vi "Move Mirror.vi"(7 "Mono System # (0)":T1, 8 "error in (no error)":errorcluster, 9 "position (side/lateral)":enum16{"side (lateral)", "front (axial)"}(ring), 10 "mirror (exit)":enum16{"entrance", "exit"}(ring)=enum."exit", 11 "VISA resource name":refnum<visa-resource-name>) -> (0 "error out":errorcluster, 3 "VISA resource name out":refnum<visa-resource-name>)   [LabVIEW 2009, in "JY-SPEX-TRIAX.lvlib"]
doc: "Moves the entrance and exit mirrors to select either the front (axial) or side (lateral) positions, respectively."
uses:
  JY-SPEX-TRIAX.lvlib
  controls.llb/Monochromator System Number.ctl
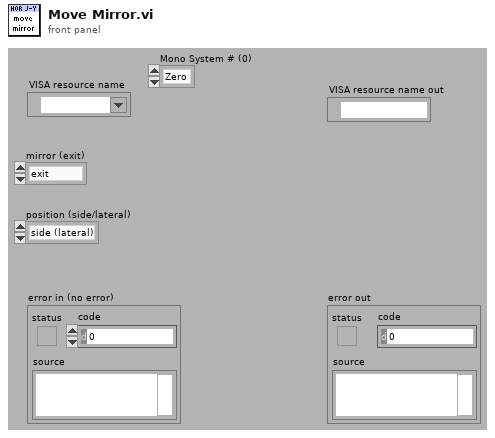
[diagram p1: front panel]
types:
  T1 = typedef "JY-SPEX-TRIAX.lvlib/Monochromator System Number.ctl" = enum16{"Zero", "One"}
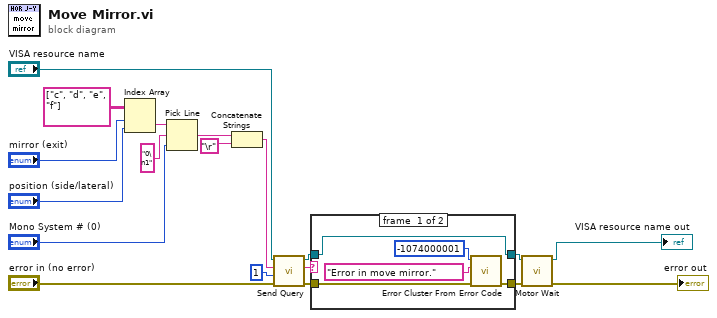
[diagram p0: block diagram]
diagram:
  n1 = Index Array(array=string[][] [["c", "d"], ["e", "f"]], index (row)="mirror (exit)", index (col)="position (side/lateral)") -> (element=w5:string)
  n2 = Pick Line(string ("")=w5, multi-line string="0\n1", line index="Mono System # (0)") -> (output string=w17:string)
  n3 = Concatenate Strings(w17, "\r") -> (w10:string)
  n4 = call "Send Query.vi"("error in (no error)"="error in (no error)", "byte count"=u32 1, "write buffer"=w10, "VISA resource name"="VISA resource name") -> ("error out"=w12:errorcluster, "read buffer"=w14:string, "VISA resource name out"=w13:refnum<visa-resource-name>)  [unwired: 5 out]
  n5 = case shown="Default" w14 {
    tunnel: w13 -> [w20 w26]
    tunnel: [w20 w26] -> w4
    tunnel: w12 -> [w22 w25]
    tunnel: [w21 w25] -> w3
    frame #0 {
      n6 = call <vilib>:"Error Cluster From Error Code.vi"("error in (no error)"=w22, "error message (\"\")"="Error in move mirror." ("error message (\"\")"), "error code (0)"=-1074000001) -> ("error out"=w21:errorcluster)  [unwired: 1 in, 5 out]
    }
    frame #1 {
    }
  }
  n7 = call "Motor Wait.vi"("error in"=w3, "VISA resource name in"=w4) -> ("error out"=→"error out":errorcluster, "VISA resource name out"=→"VISA resource name out":refnum<visa-resource-name>)  [unwired: 8 out]
